vi "live view D02.vi"() -> ()   [LabVIEW 2019, in "D02.lvlib"]
uses:
  D02.lvlib
  <vilib>/userDefined/High Color/IMAQdx.ctl
  <vilib>/vision/Image Controls.llb/IMAQ Image.ctl
  <vilib>/measure/mamon.llb/Trigger Detection for 1 Channel.vi
  <vilib>/measure/NI_MAPro.lvlib
  Calibration Lib.lvlib
  database.lvlib
  <vilib>/vision/driver/NI_Vision_Acquisition_Software.lvlib
panel:
  out "Error out":errorcluster
  in  "Save Button":bool
  in  "Calib IMQ Num":u16(ring) items=["First IMQ", "Second IMQ", "Third IMQ"]
  in  "Verify Calibration1 D02":bool caption="capture grab"
  in  "snapshot":bool
  out "error prj02":errorcluster
  in  "Verify Calibration D02":bool caption="capture grab"
  in  "Close":bool
  in  "Method 2 save D02":bool caption="capture grab"
  in  "Method 1 Save D02":bool caption="Saving txt"
  out "Average Result":string="Average Result"
  out ">18  A":dbl(slide)=1.0 caption=">16 mm" scale=0.0..100.0
  out "16-18  A":dbl(slide)=1.0 caption="14-16 mm" scale=0.0..100.0
  out "14-16  A":dbl(slide)=1.0 caption="12.7-14 mm" scale=0.0..100.0
  out "12.5-14 A":dbl(slide)=1.0 caption="11-12.7 mm" scale=0.0..100.0
  out "10-12.5  A":dbl(slide)=1.0 caption="9.5-11 mm" scale=0.0..100.0 scale format="%#_4f"
  out "8-10  A":dbl(slide)=1.0 caption="8-9.5 mm" scale=0.0..100.0
  out "6.3-8  A":dbl(slide)=1.0 caption="6.3-8 mm" scale=0.0..100.0
  out "<6.3  A":dbl(slide)=1.0 caption="<6.3 mm" scale=0.0..100.0
  out "Live Result":string="Live Result"
  out ">18  L":dbl(slide)=1.0 caption=">16 mm" scale=0.0..100.0
  out "Live View":T1(plugin-control) caption="Disc 26"
  out "16-18  L":dbl(slide)=1.0 caption="14-16 mm" scale=0.0..100.0
  out "14-16  L":dbl(slide)=1.0 caption="12.7-14 mm" scale=0.0..100.0
  out "12.5-14 L":dbl(slide)=1.0 caption="11-12.7 mm" scale=0.0..100.0
  out "10-12.5  L":dbl(slide)=1.0 caption="9.5-11 mm" scale=0.0..100.0 scale format="%#_4f"
  out "8-10  L":dbl(slide)=1.0 caption="8-9.5 mm" scale=0.0..100.0
  out "6.3-8  L":dbl(slide)=1.0 caption="6.3-8 mm" scale=0.0..100.0
  out "<6.3  L":dbl(slide)=1.0 caption="<6.3 mm" scale=0.0..100.0
  out "disc name":string="Live Info Disc 02"
  out "dsgs":string="DSGS"
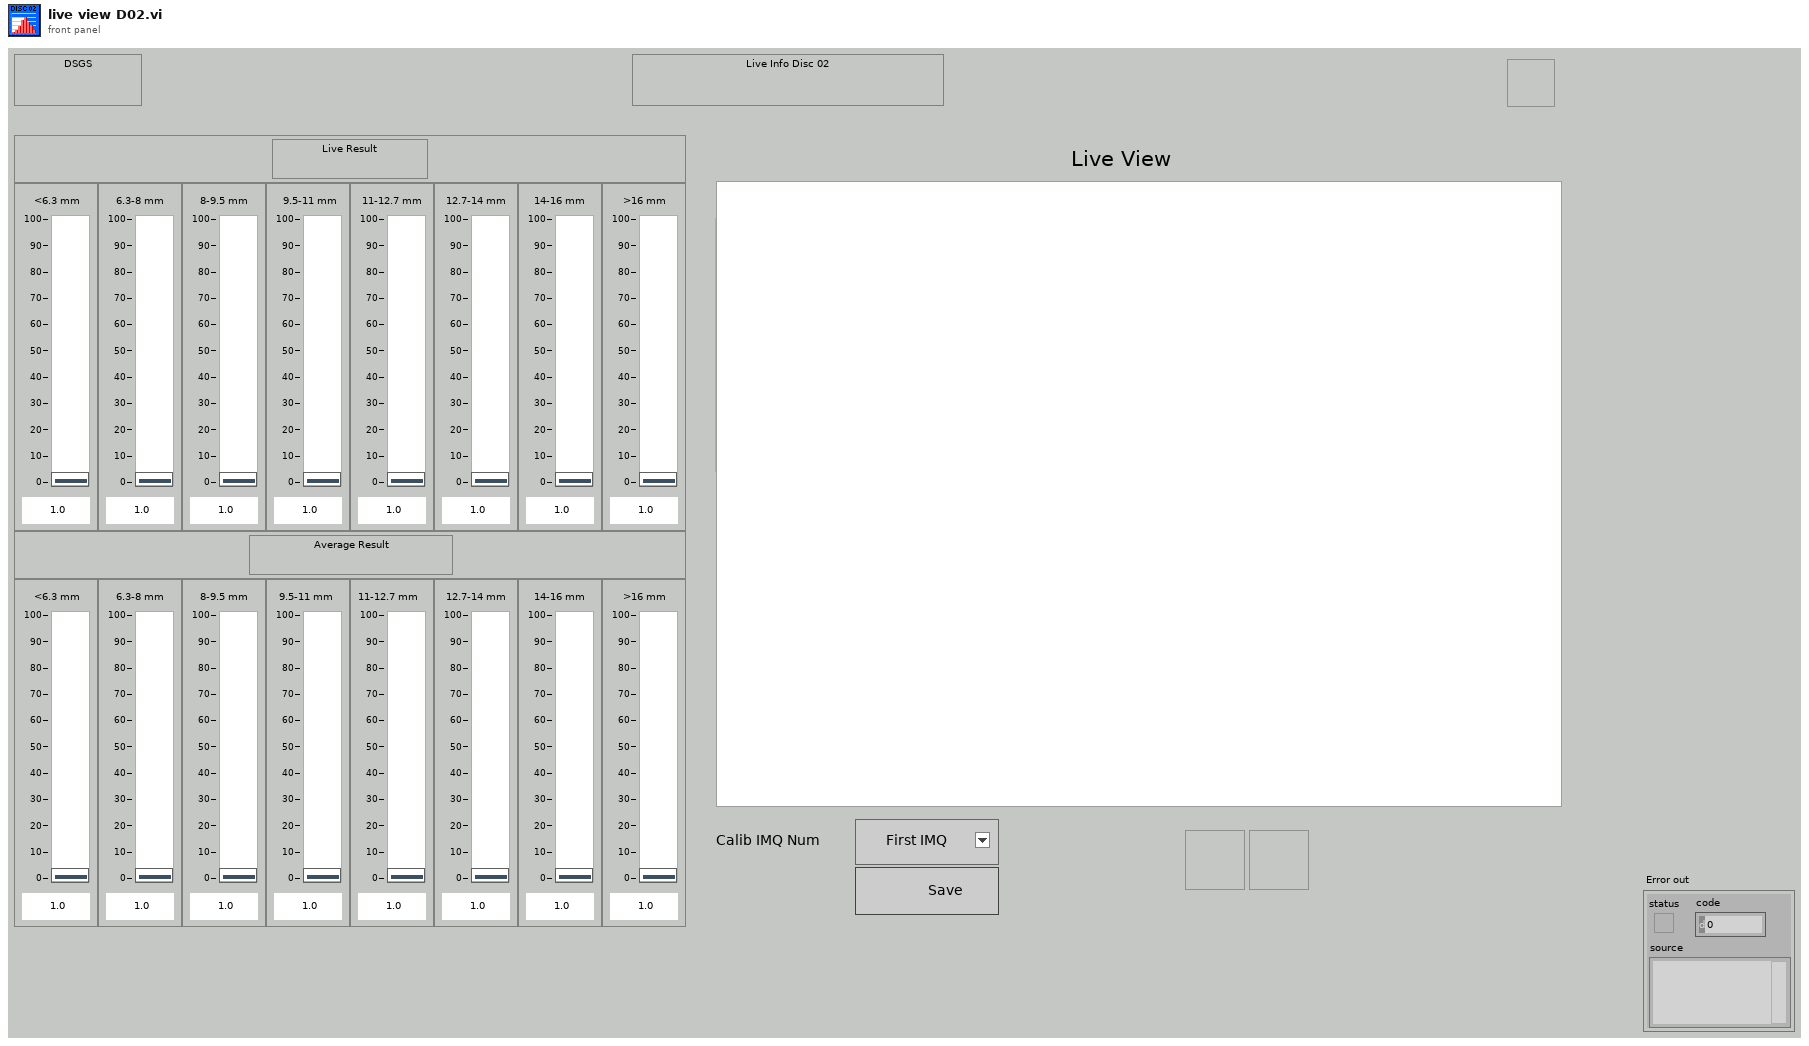
[diagram p1: front panel]
types:
  T1 = typedef "IMAQ Image.ctl" = refnum<image>
  T2 = typedef "IMAQdx.ctl" = refnum<k21>
  T3 = enum8{"Enabled", "Disabled", "Disabled and Grayed Out"}
  T4 = cluster{"date/time string":string, "date/time string":string, string, "Value":dbl, "Value":dbl, "Value":dbl, "Value":dbl, "Value":dbl, "Value":dbl, "Value":dbl, "Value":dbl}
  T5 = cluster{"date/time string":string, "date/time string":string, i32, "spreadsheet string":string, "spreadsheet string":string}
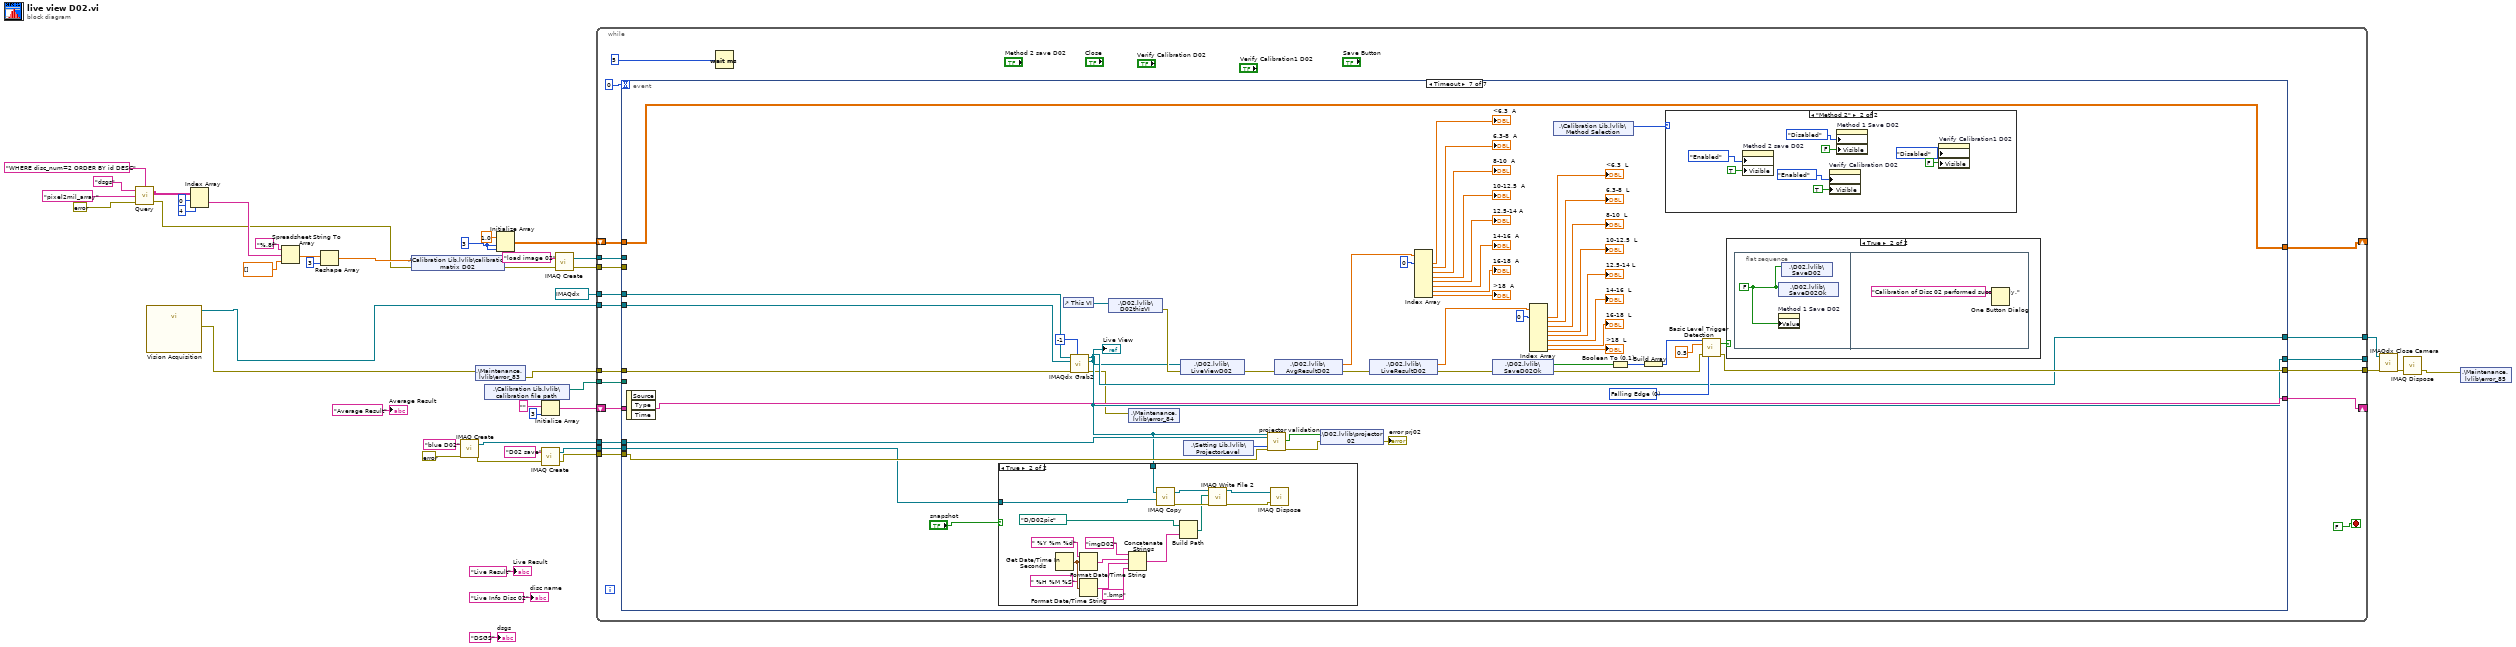
[diagram p0: block diagram]
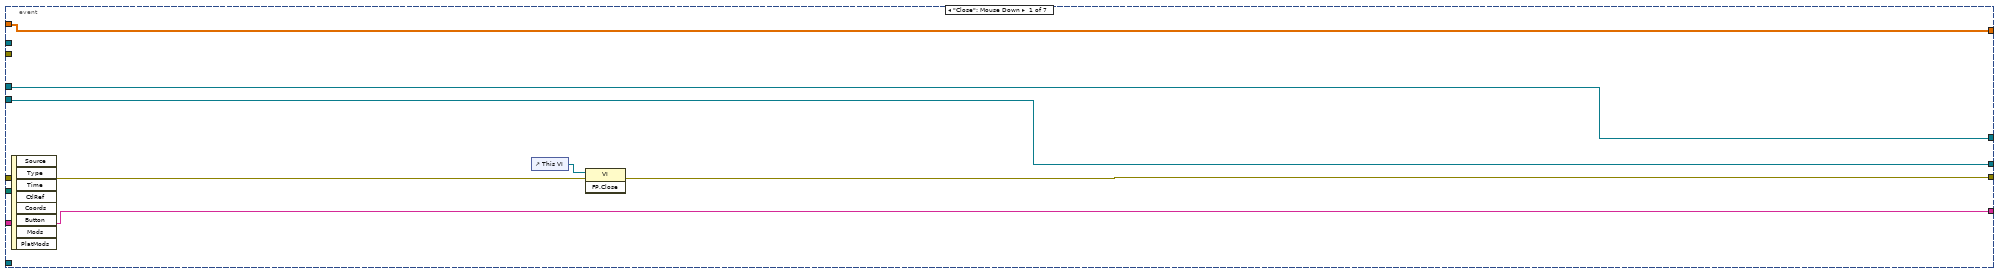
[diagram p2: hidden frame]
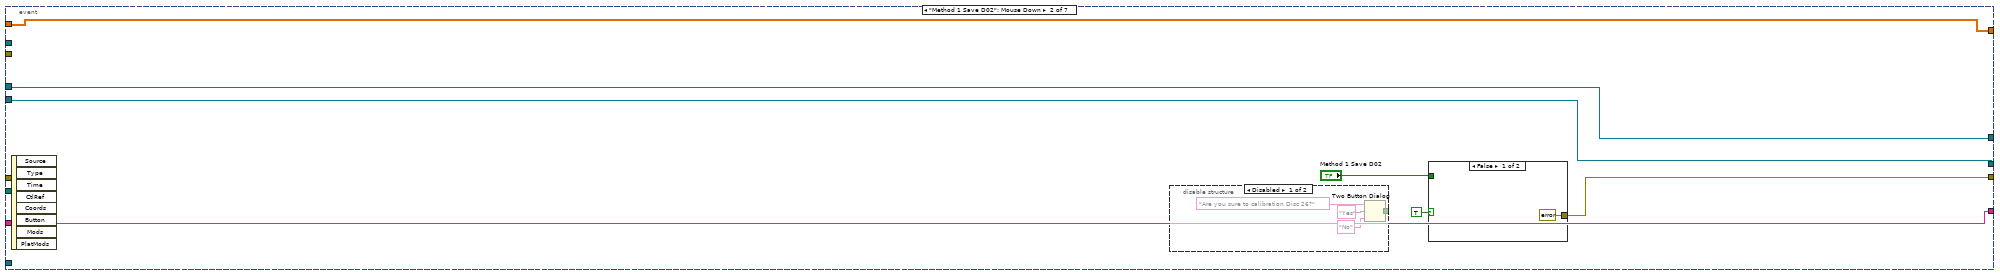
[diagram p3: hidden frame]
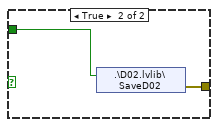
[diagram p5: hidden frame]
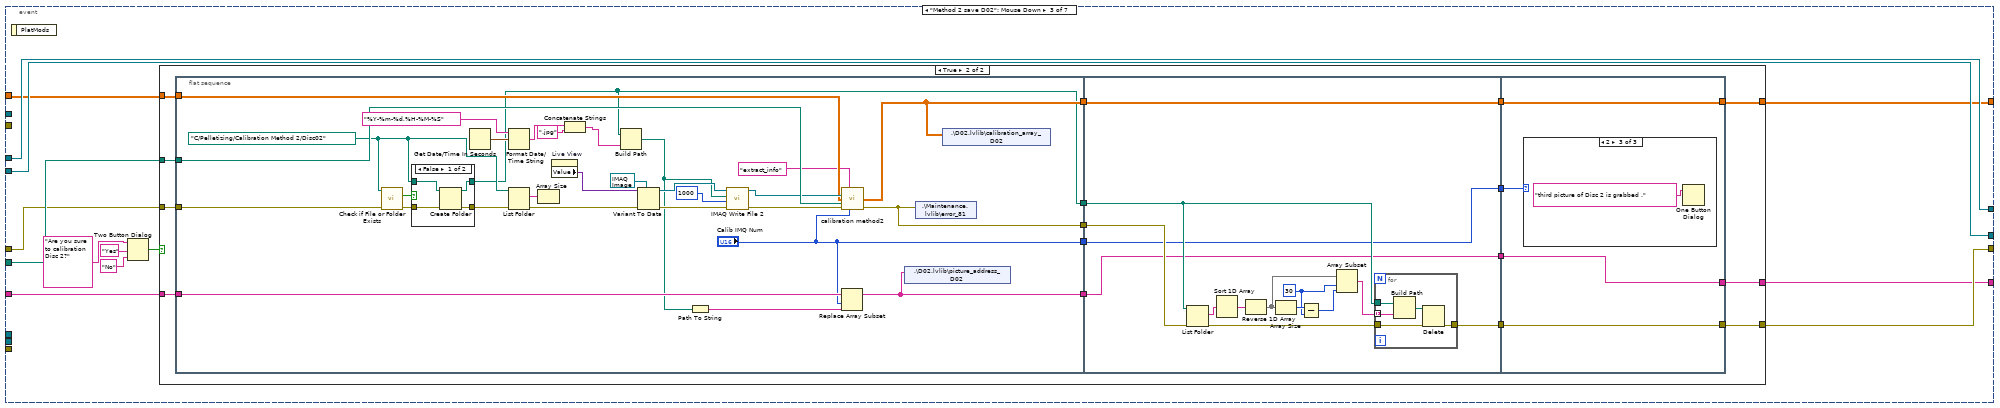
[diagram p6: hidden frame]
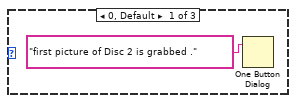
[diagram p9: hidden frame]
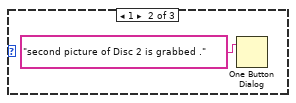
[diagram p10: hidden frame]
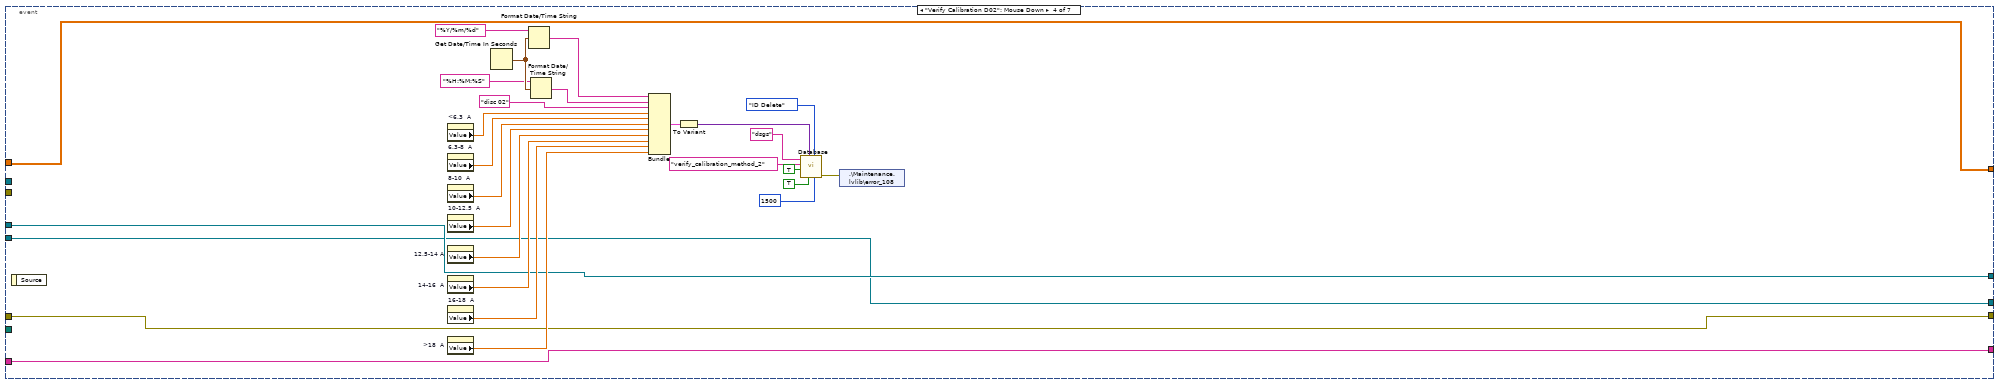
[diagram p11: hidden frame]
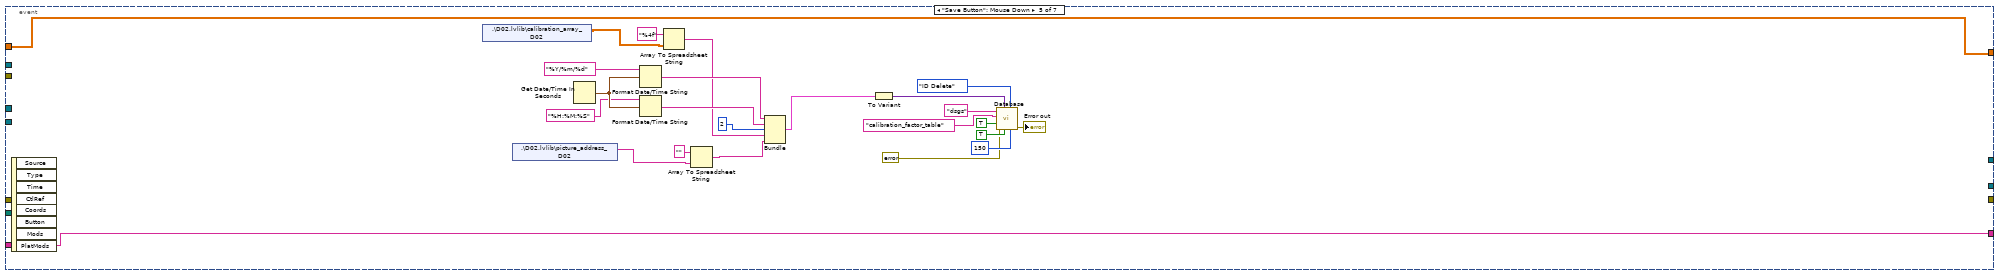
[diagram p12: hidden frame]
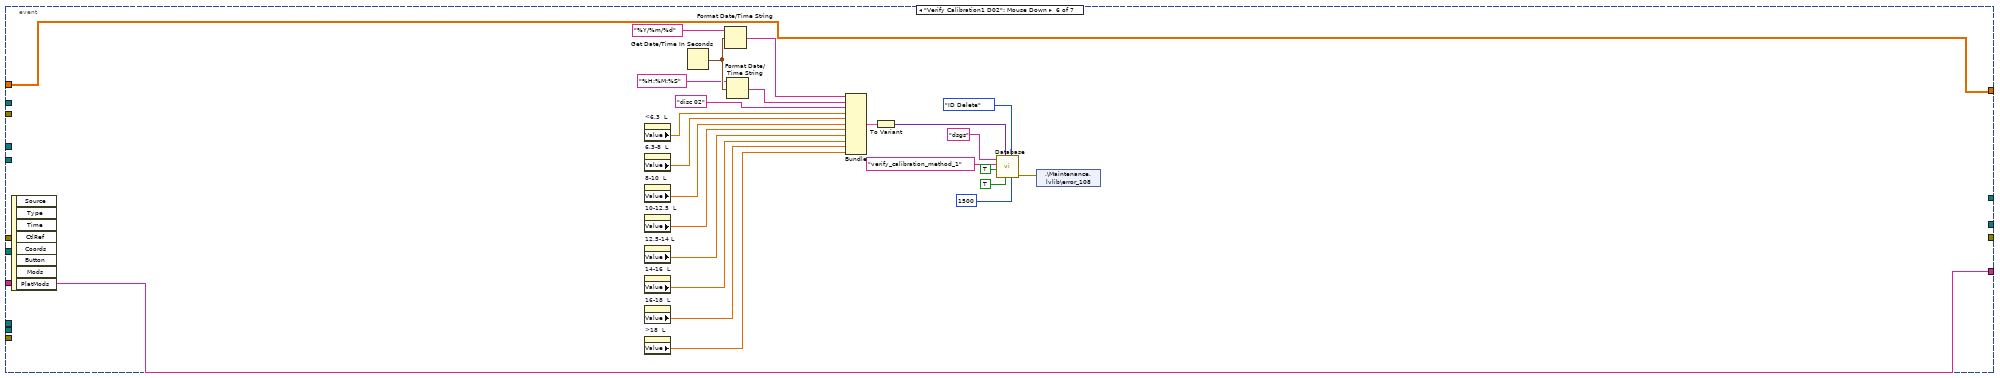
[diagram p13: hidden frame]
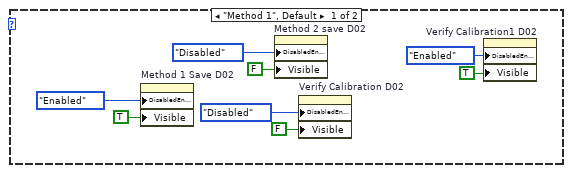
[diagram p15: hidden frame]
diagram:
  w13 = 3 ("dimension size")
  n1 = call "Query.vi"("Condition"="WHERE disc_num=2 ORDER BY id DESC", "Error in"=errorcluster {"status"=FALSE, "code"=0, "source"=""}, "Table Name"="pixel2mil_array", "Connection Name"="dsgs") -> ("Error out"=w5:errorcluster, "data"=w8:string[][])
  n2 = call "Vision Acquisition"() -> ("Image Out"=w2:T1, "error out"=w1:errorcluster)  [unwired: 25 in, 1 out]
  n3 = Index Array(array=w8, index (row)=0, index (col)=4 ("disabled index (col)")) -> (element=w6:string)
  n4 = Spreadsheet String To Array(format string="%.8f", spreadsheet string=w6, array type (2D Dbl)=sgl[] []) -> (array=w26:sgl[])  [unwired: 1 in]
  n5 = Reshape Array(w26, 3 ("dimension size")) -> (w23:sgl[])
  n6 = shared-variable ".\\Calibration Lib.lvlib\\calibration matrix D02"(w23, error in=w5) -> (error out=w22:errorcluster)
  n7 = call "IMAQ Create"("Image Name"="blue D02", "error in (no error)"=errorcluster {"status"=FALSE, "code"=0, "source"=""}) -> ("New Image"=w20:T1, "error out"=w18:errorcluster)  [unwired: 3 in]
  n8 = shared-variable ".\\Maintenance.lvlib\\error_83"(w1) -> (error out=w35:errorcluster)  [unwired: 1 in]
  n9 = shared-variable ".\\Calibration Lib.lvlib\\calibration file path"() -> (w36:path)  [unwired: 1 in, 1 out]
  n10 = Initialize Array(1.0 ("element"), w13, w13) -> (w12:dbl[][])
  n11 = call "IMAQ Create"("Image Name"="D02 save", "error in (no error)"=w18) -> ("New Image"=w15:T1, "error out"=w17:errorcluster)  [unwired: 3 in]
  n12 = Initialize Array("", 3 ("dimension size")) -> (w9:string[])
  n13 = call "IMAQ Create"("Image Name"="load image 02", "error in (no error)"=w22) -> ("New Image"=w32:T1, "error out"=w33:errorcluster)  [unwired: 3 in]
  n14 = while {
    tunnel: w36 -> [w61]
    tunnel: w35 -> [w60]
    tunnel: w2 -> [w58]
    tunnel: [w57] -> w40
    tunnel: [w56] -> _
    tunnel: T2 "cam1" ("Session In") -> [w55]
    tunnel: [w54] -> w37
    tunnel: w33 -> [w53]
    tunnel: w32 -> [w52]
    tunnel: w20 -> [w51]
    tunnel: w17 -> [w50]
    tunnel: w15 -> [w49]
    shift-right: [w47] -> _
    shift-left: w12 -> [w48]
    shift-right: [w45] -> _
    shift-left: w9 -> [w46]
    stop <- FALSE stop-if-true
    n15 = event shown="[6] Timeout" {
      selector: _ -> [_ _ _ _ _ _ _]
      dyn-events: _ -> [_ _ _ _ _ _ _]
      timeout: 0 -> [_ _ _ _ _ _ _]
      tunnel: w61 -> [_ _ w97 _ _ _ _]
      tunnel: [w69 w77 w93 w185 _ _ w274] -> w57
      tunnel: w60 -> [w68 _ w96 w185 _ _ w262]
      tunnel: w58 -> [w67 w76 w95 w183 _ _ w261]
      tunnel: [w67 w76 w95 w183 _ _ w258] -> w56
      tunnel: w55 -> [w66 w75 w94 w184 _ _ w260]
      tunnel: [w66 w75 w94 w184 _ _ w259] -> w54
      tunnel: w53 -> [_ _ _ _ _ _ _]
      tunnel: w52 -> [_ _ _ _ _ _ _]
      tunnel: w51 -> [_ _ _ _ _ _ w272]
      tunnel: w50 -> [_ _ _ _ _ _ w268]
      tunnel: w49 -> [_ _ _ _ _ _ w265]
      tunnel: w48 -> [w65 w72 w88 w180 w209 w232 w264]
      tunnel: [w65 w72 w87 w180 w209 w232 w264] -> w47
      tunnel: w46 -> [w64 w71 w86 w179 w208 w231 w263]
      tunnel: [w64 w71 w85 w179 w208 w231 w263] -> w45
      event "Close": Mouse Down {
        n16 = event-data() -> ()  [unwired: 1 in, 8 out]
        n17 = control-ref of="This VI"() -> (w70:refnum<vi>)
        n18 = invoke class="VI" method="FP.Close"(reference=w70, error in=w68) -> (error out=w69:errorcluster)  [unwired: 1 in, 2 out]
      }
      event "Method 1 Save D02": Mouse Down {
        n19 = event-data() -> ()  [unwired: 1 in, 8 out]
        n20 = disable-structure shown="Disabled" {
          disable-tunnel: [w78 _] -> _
          frame Disabled {
            n21 = Two Button Dialog(message="Are you sure to calibration Disc 26?", 1:"No" ("F button name (\"Cancel\")"), 2:"Yes" ("T button name (\"OK\")")) -> (T button?=w78:bool)
          }
          frame Enabled {
          }
        }
        n22 = case shown="False" TRUE {
          tunnel: [errorcluster {"status"=FALSE, "code"=0, "source"=""} ("error IO") w84] -> w77
          tunnel: "Method 1 Save D02" -> [_ w83]
          frame False {
          }
          frame True {
            n23 = shared-variable ".\\D02.lvlib\\SaveD02"(w83) -> (error out=w84:errorcluster)  [unwired: 1 in]
          }
        }
      }
      event "Method 2 save D02": Mouse Down {
        n24 = event-data() -> ()  [unwired: 1 in, 1 out]
        n25 = Two Button Dialog(message="Are you sure to calibration Disc 2?", 1:"No" ("F button name (\"Cancel\")"), 2:"Yes" ("T button name (\"OK\")")) -> (T button?=w89:bool)
        n26 = case shown="True" w89 {
          tunnel: w97 -> [_ w115]
          tunnel: w96 -> [w100 w114]
          tunnel: [w100 w113] -> w93
          tunnel: w88 -> [w99 w111]
          tunnel: [w99 w108] -> w87
          tunnel: w86 -> [w98 w107]
          tunnel: [w98 w104] -> w85
          frame False {
          }
          frame True {
            n27 = flat-sequence {
              tunnel: w114 -> [w135]
              tunnel: w115 -> [w146]
              tunnel: [w121] -> w116
              tunnel: w111 -> [w128]
              tunnel: [w127] -> w109
              tunnel: w107 -> [w124]
              tunnel: [w123] -> w105
              tunnel: [w122] -> w103
              tunnel: ["Calib IMQ Num"] -> w101
              tunnel: [w157] -> w112
              tunnel: [w155] -> w110
              tunnel: [w154] -> w106
              tunnel: w103 -> [w158]
              tunnel: w105 -> [w154]
              tunnel: w109 -> [w155]
              tunnel: w116 -> [w159]
              tunnel: [w153] -> w102
              tunnel: w101 -> [w153]
              tunnel: [w175] -> w113
              tunnel: w112 -> [w175]
              tunnel: [w174] -> w108
              tunnel: w110 -> [w174]
              tunnel: [w173] -> w104
              tunnel: w106 -> [w173]
              tunnel: w102 -> [w172]
              frame #0 {
                w131 = path "C:/Pelletizing/Calibration Method 2/Disc02" ("path")
                n28 = call <vilib>:"Check if File or Folder Exists.vi"("error in (no error)"=w135, "path"=w131) -> ("error out"=w136:errorcluster, "file or folder exists?"=w137:bool)  [unwired: 7 in, 1 out]
                n29 = case shown="False" w137 {
                  tunnel: [w148 w152] -> w121
                  tunnel: w131 -> [w150 w152]
                  tunnel: w136 -> [w149 w151]
                  tunnel: [w147 w151] -> w133
                  frame False {
                    n30 = Create Folder(path (use dialog)=w150, error in=w149) -> (created path=w148:path, error out=w147:errorcluster)  [unwired: 1 in, 1 out]
                  }
                  frame True {
                  }
                }
                n31 = Get Date/Time In Seconds() -> (seconds since 1Jan1904=w141:timestamp)
                n32 = Format Date/Time String(time format string (%c)="%Y-%m-%d,%H-%M-%S", seconds (now)=w141) -> (date/time string=w139:string)  [unwired: 1 in]
                n33 = List Folder(path=w131, error in=w133) -> (filenames=w134:string[], error out=w132:errorcluster)  [unwired: 2 in, 2 out]
                n34 = Array Size(array=w134) -> ()  [unwired: 1 out]
                n35 = property on="Live View" class="ImageControl"() -> ("Value"=w145:variant)  [unwired: 2 in, 2 out]
                n36 = Concatenate Strings(w139, ".jpg" ("string")) -> (w120:string)
                n37 = Build Path(base path=w121, name or relative path=w120) -> (appended path=w119:path)
                n38 = Variant To Data(error in=w132, type=T1 refnum ("New Image"), Variant=w145) -> (data=w129:T1, error out=w142:errorcluster)
                n39 = Path To String(path=w119) -> (string=w118:string)
                n40 = call-poly "IMAQ Write File 2"("error in (no error)"=w142, "Image Quality"=u32 1000, "File Path"=w119, "Image"=w129) -> ("error out"=w126:errorcluster, "Image Out (duplicate)"=w130:T1)  [unwired: 6 in]
                n41 = Replace Array Subset(array=w124, new element=w118, index="Calib IMQ Num") -> (w123:string[])
                n42 = call "calibration method2.vi"("function name"="extract_info", "Image IN"=w130, "initialize matrix"=w128, "module path"=w146, "error in"=w126, "snap number"="Calib IMQ Num") -> ("calibration matrix"=w127:dbl[][], "error out"=w122:errorcluster)  [unwired: 8 in]
                n43 = shared-variable ".\\D02.lvlib\\picture_address_D02"(w123) -> ()  [unwired: 1 in, 1 out]
                n44 = shared-variable ".\\Maintenance.lvlib\\error_81"(w122) -> ()  [unwired: 1 in, 1 out]
                n45 = shared-variable ".\\D02.lvlib\\calibration_array_D02"(w127) -> ()  [unwired: 1 in, 1 out]
              }
              frame #1 {
                w160 = 30 ("index")
                n46 = List Folder(path=w159, error in=w158) -> (filenames=w166:string[], error out=w156:errorcluster)  [unwired: 2 in, 2 out]
                n47 = Sort 1D Array(array=w166) -> (sorted array=w165:string[])
                n48 = Reverse 1D Array(array=w165) -> (reversed array=w164:string[])
                n49 = Array Size(array=w164) -> (size(s)=w163:i32)
                n50 = Subtract(x=w163, y=w160) -> (x-y=w162:i32)
                n51 = Array Subset(array=w164, index=w160, length=w162) -> (w161:string[])
                n52 = for {
                  tunnel: w161 -> [w170] mode=indexing
                  tunnel: w159 -> [w171]
                  tunnel: [w168] -> w157
                  tunnel: w156 -> [w167]
                  n53 = Build Path(base path=w171, name or relative path=w170) -> (appended path=w169:path)
                  n54 = Delete(path (use dialog)=w169, error in=w167) -> (error out=w168:errorcluster)  [unwired: 3 in, 2 out]
                }
              }
              frame #2 {
                n55 = case shown="2" w172 {
                  frame 0, Default {
                    n56 = One Button Dialog(message="first picture of Disc 2 is grabbed .") -> ()  [unwired: 1 in, 1 out]
                  }
                  frame 1 {
                    n57 = One Button Dialog(message="second picture of Disc 2 is grabbed .") -> ()  [unwired: 1 in, 1 out]
                  }
                  frame 2 {
                    n58 = One Button Dialog(message="third picture of Disc 2 is grabbed .") -> ()  [unwired: 1 in, 1 out]
                  }
                }
              }
            }
          }
        }
      }
      event "Verify Calibration D02": Mouse Down {
        n59 = event-data() -> ()  [unwired: 1 in, 1 out]
        n60 = property on="<6.3  A" class="Slide (strict)"() -> ("Value"=w200:dbl)  [unwired: 2 in, 2 out]
        n61 = property on="6.3-8  A" class="Slide (strict)"() -> ("Value"=w199:dbl)  [unwired: 2 in, 2 out]
        n62 = property on="8-10  A" class="Slide (strict)"() -> ("Value"=w198:dbl)  [unwired: 2 in, 2 out]
        n63 = property on="10-12.5  A" class="Slide (strict)"() -> ("Value"=w197:dbl)  [unwired: 2 in, 2 out]
        n64 = property on="12.5-14 A" class="Slide (strict)"() -> ("Value"=w196:dbl)  [unwired: 2 in, 2 out]
        n65 = property on="14-16  A" class="Slide (strict)"() -> ("Value"=w195:dbl)  [unwired: 2 in, 2 out]
        n66 = property on="16-18  A" class="Slide (strict)"() -> ("Value"=w194:dbl)  [unwired: 2 in, 2 out]
        n67 = property on=">18  A" class="Slide (strict)"() -> ("Value"=w193:dbl)  [unwired: 2 in, 2 out]
        n68 = Get Date/Time In Seconds() -> (seconds since 1Jan1904=w205:timestamp)
        n69 = Format Date/Time String(time format string (%c)="%Y/%m/%d", seconds (now)=w205) -> (date/time string=w203:string)  [unwired: 1 in]
        n70 = Format Date/Time String(time format string (%c)="%H:%M:%S", seconds (now)=w205) -> (date/time string=w202:string)  [unwired: 1 in]
        n71 = Bundle("date/time string"=w203, "date/time string"=w202, "disc 02", "Value"=w200, "Value"=w199, "Value"=w198, "Value"=w197, "Value"=w196, "Value"=w195, "Value"=w194, "Value"=w193) -> (w192:T4)  [unwired: 1 in]
        n72 = To Variant(anything=w192) -> (Variant=w191:variant)
        n73 = call "Database.vi"("Maximum Row"=1500, "Enum"=enum16{"ID Delete", "Time Delete"}."ID Delete", "Delete row?"=TRUE, "Data"=w191, "Auto Increment ID?"=TRUE, "Table"="verify_calibration_method_2", "Connection"="dsgs") -> ("Error out"=w186:errorcluster)  [unwired: 4 in]
        n74 = shared-variable ".\\Maintenance.lvlib\\error_108"(w186) -> ()  [unwired: 1 in, 1 out]
      }
      event "Save Button": Mouse Down {
        n75 = event-data() -> ()  [unwired: 1 in, 8 out]
        n76 = shared-variable ".\\D02.lvlib\\calibration_array_D02"() -> (w210:dbl[][])  [unwired: 1 in, 1 out]
        n77 = shared-variable ".\\D02.lvlib\\picture_address_D02"() -> (w212:string[])  [unwired: 1 in, 1 out]
        n78 = Get Date/Time In Seconds() -> (seconds since 1Jan1904=w219:timestamp)
        n79 = Format Date/Time String(time format string (%c)="%Y/%m/%d", seconds (now)=w219) -> (date/time string=w220:string)  [unwired: 1 in]
        n80 = Format Date/Time String(time format string (%c)="%H:%M:%S", seconds (now)=w219) -> (date/time string=w218:string)  [unwired: 1 in]
        n81 = Array To Spreadsheet String(array=w210, 3:"%4f" ("format string")) -> (spreadsheet string=w214:string)  [unwired: 1 in]
        n82 = Array To Spreadsheet String(array=w212, 3:"" ("format string")) -> (spreadsheet string=w211:string)  [unwired: 1 in]
        n83 = Bundle("date/time string"=w220, "date/time string"=w218, 2, "spreadsheet string"=w214, "spreadsheet string"=w211) -> (w223:T5)  [unwired: 1 in]
        n84 = To Variant(anything=w223) -> (Variant=w230:variant)
        n85 = call "Database.vi"("Maximum Row"=150, "Enum"=enum16{"ID Delete", "Time Delete"}."ID Delete", "Delete row?"=TRUE, "Data"=w230, "Error in"=errorcluster {"status"=FALSE, "code"=0, "source"=""}, "Auto Increment ID?"=TRUE, "Table"="calibration_factor_table", "Connection"="dsgs") -> ("Error out"=→"Error out":errorcluster)  [unwired: 3 in]
      }
      event "Verify Calibration1 D02": Mouse Down {
        n86 = event-data() -> ()  [unwired: 1 in, 8 out]
        n87 = property on="<6.3  L" class="Slide (strict)"() -> ("Value"=w249:dbl)  [unwired: 2 in, 2 out]
        n88 = property on="6.3-8  L" class="Slide (strict)"() -> ("Value"=w248:dbl)  [unwired: 2 in, 2 out]
        n89 = property on="8-10  L" class="Slide (strict)"() -> ("Value"=w247:dbl)  [unwired: 2 in, 2 out]
        n90 = property on="10-12.5  L" class="Slide (strict)"() -> ("Value"=w246:dbl)  [unwired: 2 in, 2 out]
        n91 = property on="12.5-14 L" class="Slide (strict)"() -> ("Value"=w245:dbl)  [unwired: 2 in, 2 out]
        n92 = property on="14-16  L" class="Slide (strict)"() -> ("Value"=w244:dbl)  [unwired: 2 in, 2 out]
        n93 = property on="16-18  L" class="Slide (strict)"() -> ("Value"=w243:dbl)  [unwired: 2 in, 2 out]
        n94 = property on=">18  L" class="Slide (strict)"() -> ("Value"=w242:dbl)  [unwired: 2 in, 2 out]
        n95 = Get Date/Time In Seconds() -> (seconds since 1Jan1904=w254:timestamp)
        n96 = Format Date/Time String(time format string (%c)="%Y/%m/%d", seconds (now)=w254) -> (date/time string=w252:string)  [unwired: 1 in]
        n97 = Format Date/Time String(time format string (%c)="%H:%M:%S", seconds (now)=w254) -> (date/time string=w251:string)  [unwired: 1 in]
        n98 = Bundle("date/time string"=w252, "date/time string"=w251, "disc 02", "Value"=w249, "Value"=w248, "Value"=w247, "Value"=w246, "Value"=w245, "Value"=w244, "Value"=w243, "Value"=w242) -> (w241:T4)  [unwired: 1 in]
        n99 = To Variant(anything=w241) -> (Variant=w240:variant)
        n100 = call "Database.vi"("Maximum Row"=1500, "Enum"=enum16{"ID Delete", "Time Delete"}."ID Delete", "Delete row?"=TRUE, "Data"=w240, "Auto Increment ID?"=TRUE, "Table"="verify_calibration_method_1", "Connection"="dsgs") -> ("Error out"=w235:errorcluster)  [unwired: 4 in]
        n101 = shared-variable ".\\Maintenance.lvlib\\error_108"(w235) -> ()  [unwired: 1 in, 1 out]
      }
      event Timeout {
        w282 = u16 0 items=["Falling Edge", "Rising Edge"] ("trigger slope")
        n102 = event-data() -> ()  [unwired: 1 in, 3 out]
        n103 = control-ref of="This VI"() -> (w277:refnum<vi>)
        n104 = call <vilib>:"IMAQdx Grab2.vi"("Timeout (ms)"=-1, "error in"=w262, "Image In"=w261, "Session In"=w260) -> ("error out"=w257:errorcluster, "Image Out"=w258:T1, "Session Out"=w259:T2)  [unwired: 4 in, 1 out]
        "Live View" <- w258
        n105 = case shown="True" "snapshot" {
          tunnel: w265 -> [_ w322]
          tunnel: w258 -> [_ w321]
          frame False {
          }
          frame True {
            n106 = Get Date/Time In Seconds() -> (seconds since 1Jan1904=w315:timestamp)
            n107 = Format Date/Time String(time format string (%c)=" %Y %m %d", seconds (now)=w315) -> (date/time string=w311:string)  [unwired: 1 in]
            n108 = Format Date/Time String(time format string (%c)=" %H %M %S", seconds (now)=w315) -> (date/time string=w310:string)  [unwired: 1 in]
            n109 = Concatenate Strings("imgD02" ("string"), w311, w310, ".bmp" ("string")) -> (w308:string)
            n110 = call "IMAQ Copy"("Image Dst"=w322, "Image Src"=w321) -> ("error out"=w319:errorcluster, "Image Dst Out"=w320:T1)  [unwired: 4 in]
            n111 = Build Path(base path=path "D:/D02pic" ("File Path"), name or relative path=w308) -> (appended path=w307:path)
            n112 = call-poly "IMAQ Write File 2"("error in (no error)"=w319, "File Path"=w307, "Image"=w320) -> ("error out"=w317:errorcluster, "Image Out (duplicate)"=w318:T1)  [unwired: 7 in]
            n113 = call "IMAQ Dispose"("Image"=w318, "error in (no error)"=w317) -> ()  [unwired: 4 in, 1 out]
          }
        }
        n114 = shared-variable ".\\D02.lvlib\\D02thisVI"(w277) -> (error out=w273:errorcluster)  [unwired: 1 in]
        n115 = shared-variable ".\\Maintenance.lvlib\\error_84"(w257) -> ()  [unwired: 1 in, 1 out]
        n116 = shared-variable ".\\D02.lvlib\\LiveViewD02"(w258, error in=w273) -> (error out=w276:errorcluster)
        n117 = shared-variable ".\\Setting Lib.lvlib\\ProjectorLevel"() -> (w267:i32)  [unwired: 1 in, 1 out]
        n118 = call "projector validation.vi"("Image Src"=w258, "blue channel"=w272, "on/off level"=w267, "error in (no error)"=w268) -> ("on/off"=w271:bool, "error out"=w270:errorcluster)  [unwired: 14 in]
        n119 = shared-variable ".\\D02.lvlib\\AvgResultD02"(error in=w276) -> (w297:dbl[], error out=w279:errorcluster)
        n120 = shared-variable ".\\D02.lvlib\\projector 02"(w271, error in=w270) -> (error out=→"error prj02":errorcluster)
        n121 = shared-variable ".\\D02.lvlib\\LiveResultD02"(error in=w279) -> (w296:dbl[], error out=w278:errorcluster)
        n122 = Index Array(array=w297, index #1=0 ("index")) -> (element #1=→"<6.3  A":dbl, element #2=→"6.3-8  A":dbl, element #3=→"8-10  A":dbl, element #4=→"10-12.5  A":dbl, element #5=→"12.5-14 A":dbl, element #6=→"14-16  A":dbl, element #7=→"16-18  A":dbl, element #8=→">18  A":dbl)  [unwired: 7 in]
        n123 = shared-variable ".\\D02.lvlib\\SaveD02Ok"(error in=w278) -> (w283:bool, error out=w275:errorcluster)
        n124 = Index Array(array=w296, index #1=0 ("index")) -> (element #1=→"<6.3  L":dbl, element #2=→"6.3-8  L":dbl, element #3=→"8-10  L":dbl, element #4=→"10-12.5  L":dbl, element #5=→"12.5-14 L":dbl, element #6=→"14-16  L":dbl, element #7=→"16-18  L":dbl, element #8=→">18  L":dbl)  [unwired: 7 in]
        n125 = shared-variable ".\\Calibration Lib.lvlib\\Method Selection"() -> (w280:enum32{"Method 1", "Method 2"})  [unwired: 1 in, 1 out]
        n126 = Boolean To (0,1)(Boolean=w283) -> (0, 1=w286:i16)
        n127 = Build Array(w286) -> (w285:i16[])
        n128 = case shown="\"Method 2\"" w280 {
          frame "Method 1", Default {
            n129 = property on="Method 1 Save D02" class="Bool (strict)"("DisabledEnum"=T3."Enabled" ("Disabled"), "Visible"=TRUE) -> ()  [unwired: 2 in, 2 out]
            n130 = property on="Method 2 save D02" class="Bool (strict)"("DisabledEnum"=T3."Disabled" ("Disabled"), "Visible"=FALSE) -> ()  [unwired: 2 in, 2 out]
            n131 = property on="Verify Calibration D02" class="Bool (strict)"("DisabledEnum"=T3."Disabled" ("Disabled"), "Visible"=FALSE) -> ()  [unwired: 2 in, 2 out]
            n132 = property on="Verify Calibration1 D02" class="Bool (strict)"("DisabledEnum"=T3."Enabled" ("Disabled"), "Visible"=TRUE) -> ()  [unwired: 2 in, 2 out]
          }
          frame "Method 2" {
            n133 = property on="Method 2 save D02" class="Bool (strict)"("DisabledEnum"=T3."Enabled" ("Disabled"), "Visible"=TRUE) -> ()  [unwired: 2 in, 2 out]
            n134 = property on="Verify Calibration D02" class="Bool (strict)"("DisabledEnum"=T3."Enabled" ("Disabled"), "Visible"=TRUE) -> ()  [unwired: 2 in, 2 out]
            n135 = property on="Method 1 Save D02" class="Bool (strict)"("DisabledEnum"=T3."Disabled" ("Disabled"), "Visible"=FALSE) -> ()  [unwired: 2 in, 2 out]
            n136 = property on="Verify Calibration1 D02" class="Bool (strict)"("DisabledEnum"=T3."Disabled" ("Disabled"), "Visible"=FALSE) -> ()  [unwired: 2 in, 2 out]
          }
        }
        n137 = call-poly <vilib>:"Basic Level Trigger Detection.vi"("signal in"=w285, "level"=0.5, "error in (no error)"=w275, "trigger slope"=w282) -> ("trigger detected?"=w281:bool, "error out"=w274:errorcluster)  [unwired: 9 in, 1 out]
        n138 = case shown="True" w281 {
          frame False {
          }
          frame True {
            n139 = flat-sequence {
              frame #0 {
                w339 = FALSE
                n140 = shared-variable ".\\D02.lvlib\\SaveD02Ok"(w339) -> ()  [unwired: 1 in, 1 out]
                n141 = property on="Method 1 Save D02" class="Bool (strict)"("Value"=w339) -> ()  [unwired: 2 in, 2 out]
                n142 = shared-variable ".\\D02.lvlib\\SaveD02"(w339) -> ()  [unwired: 1 in, 1 out]
              }
              frame #1 {
                n143 = One Button Dialog(message="Calibration of Disc 02 performed successfully.") -> ()  [unwired: 1 in, 1 out]
              }
            }
          }
        }
      }
    }
    n144 = Wait (ms)(milliseconds to wait=u32 5) -> ()  [unwired: 1 out]
  }
  n145 = call <vilib>:"IMAQdx Close Camera.vi"("error in"=w40, "Session In"=w37) -> ("error out"=w39:errorcluster)  [unwired: 9 in]
  n146 = call "IMAQ Dispose"("error in (no error)"=w39) -> ("error out"=w3:errorcluster)  [unwired: 5 in]
  n147 = shared-variable ".\\Maintenance.lvlib\\error_85"(w3) -> ()  [unwired: 1 in, 1 out]
  "Live Result" <- "Live Result" ("Live Result")
  "Average Result" <- "Average Result" ("Average Result")
  "disc name" <- "Live Info Disc 02" ("Live Result")
  "dsgs" <- "DSGS" ("Live Result")
